vi "Create Timestamp.vi"(8 "error in (no error)":errorcluster, 10 "Channel Paramters":T2, 11 "Message Channels Section in":T1 format="%.0x") -> (0 "error out":errorcluster, 2 "Channel Ref":T1 format="%.0x", 3 "Message Channels Section out":T1 format="%.0x")   [LabVIEW 2020, in "Instrument Addon Scripting API.lvlib"]
uses:
  Instrument Addon Scripting API.lvlib
  <vilib>/NI VeriStand/Custom Device API/Custom Device Channel.ctl
  <vilib>/NI VeriStand/Custom Device API/Custom Device Channel Type.ctl
  <vilib>/NI VeriStand/Custom Device API/Custom Device Item Ref.ctl
  Addon/Addon Shared/SubVIs/Constants.vi
  Addon/Addon Shared/Instrument Addon Shared.lvlib
  <vilib>/NI VeriStand/Custom Device API/Custom Device API.lvlib
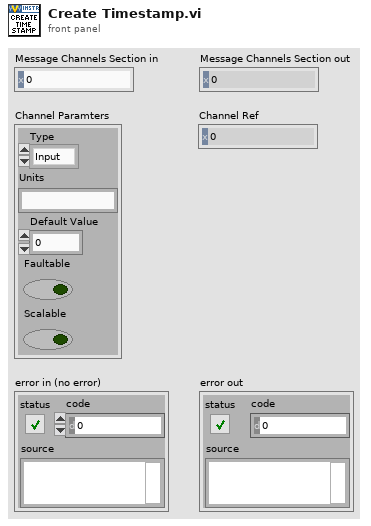
[diagram p1: front panel]
types:
  T1 = typedef "Custom Device API.lvlib/Custom Device Item Ref.ctl" = u64
  T2 = typedef "Custom Device API.lvlib/Custom Device Channel.ctl" = cluster{"Type":T3, "Units":string, "Default Value":dbl, "Faultable":bool, "Scalable":bool}
  T3 = typedef "Custom Device API.lvlib/Custom Device Channel Type.ctl" = enum16{"Input", "Output"}
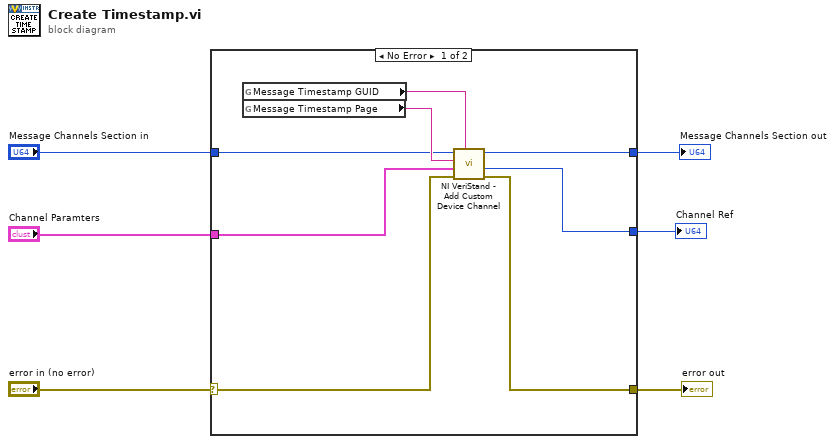
[diagram p0: block diagram]
diagram:
  n1 = case shown="No Error" "error in (no error)" {
    selector: "error in (no error)" -> [w7 w16]
    tunnel: "Channel Paramters" -> [w14 _]
    tunnel: [w13 w15] -> w5
    tunnel: [w12 w16] -> w4
    tunnel: "Message Channels Section in" -> [w9 w15]
    tunnel: [w8 _] -> w2
    frame No Error {
      n2 = global read "Constants.vi" "Message Timestamp GUID"() -> (w10:string)
      n3 = global read "Constants.vi" "Message Timestamp Page"() -> (w11:string)
      n4 = call <vilib>:"NI VeriStand - Add Custom Device Channel.vi"("GUID (Default Channel)"=w10, "error in (no error)"=w7, "Channel"=w14, "Channel Name"=w11, "Parent Ref in"=w9) -> ("error out"=w12:errorcluster, "Channel Ref"=w8:T1, "Parent Ref out"=w13:T1)  [unwired: 3 in, 1 out]
    }
    frame Error {
    }
  }
  "Message Channels Section out" <- w5
  "error out" <- w4
  "Channel Ref" <- w2
